vi "rechts.vi"   [LabVIEW 2019]
uses:
  <vilib>/myRIO/Common/Instrument Driver Framework/Utilities/typedefs/Analog Scaling Constants.ctl
  <vilib>/myRIO/Common/Instrument Driver Framework/Utilities/typedefs/Analog Scaling Constants List.ctl
  <vilib>/myRIO/Common/Instrument Driver Framework/myRIO v1.0/AO/typedefs/AO Channels Enum.ctl
  <vilib>/myRIO/Common/Instrument Driver Framework/myRIO v1.0/AO/typedefs/AO Channels List.ctl
  <vilib>/myRIO/Common/Instrument Driver Framework/Utilities/typedefs/Generic FPGA Reference.ctl
  <vilib>/myRIO/Common/Instrument Driver Framework/Utilities/typedefs/myRIO v1.0 Reference.ctl
  <vilib>/myRIO/Common/Instrument Driver Framework/Utilities/typedefs/Hardware Version Enum.ctl
  <vilib>/myRIO/Common/Instrument Driver Framework/Utilities/typedefs/myRIO Generic Hardware Reference.ctl
  <vilib>/myRIO/Instrument Drivers/Onboard IO/AO/typedefs/AO Reference.ctl
  <vilib>/myRIO/Instrument Drivers/Onboard IO/AO/AO.lvlib
  <vilib>/myRIO/Instrument Drivers/Onboard IO/AO/vis/Write.vi
  <vilib>/userDefined/High Color/nirio_resource_hc.ctl
  <vilib>/myRIO/Common/Instrument Driver Framework/myRIO v1.0/AO/vis/myRIO v1.1 Open AO.vi
  <vilib>/myRIO/Instrument Drivers/Onboard IO/AO/vis/myRIO AO Open.xnode
  <vilib>/myRIO/Common/Instrument Driver Framework/Utilities/vis/Is FPGA Ref Available.vi
  <vilib>/myRIO/Express VI/Onboard IO/AO/AO Express VI.xnode
  interface.vi
types:
  T1 = typedef "AO.lvlib/AO Reference.ctl" = cluster{"myRIO Reference":T2, "AO Channel List":T6, "AO Scaling Constant List":T8}
  T2 = typedef "myRIO Generic Hardware Reference.ctl" = cluster{"myRIO Model":T3, "myRIO Hardware Reference":T4}
  T3 = typedef "Hardware Version Enum.ctl" = enum16{"Unknown", "myRIO-1900", "myRIO-1950", "roboRIO", "NI ELVIS RIO CM", "ELVIS III"}
  T4 = typedef "myRIO v1.0 Reference.ctl" = cluster{"Generic FPGA Reference":T5, "Allow multiple opens":bool}
  T5 = typedef "Generic FPGA Reference.ctl" = refnum<k20>
  T6 = typedef "AO Channels List.ctl" = T7[]
  T7 = typedef "AO Channels Enum.ctl" = enum16{"Not Connected", "AudioOut/Left", "AudioOut/Right", "C/AO0", "C/AO1", "A/AO0", "A/AO1", "B/AO0", "B/AO1"}
  T8 = typedef "Analog Scaling Constants List.ctl" = T9[]
  T9 = typedef "Analog Scaling Constants.ctl" = cluster{"LSB Weight (Volts)":dbl, "Offset (Volts)":dbl, "Signed?":bool}
  T10 = typedef "nirio_resource_hc.ctl" = tag
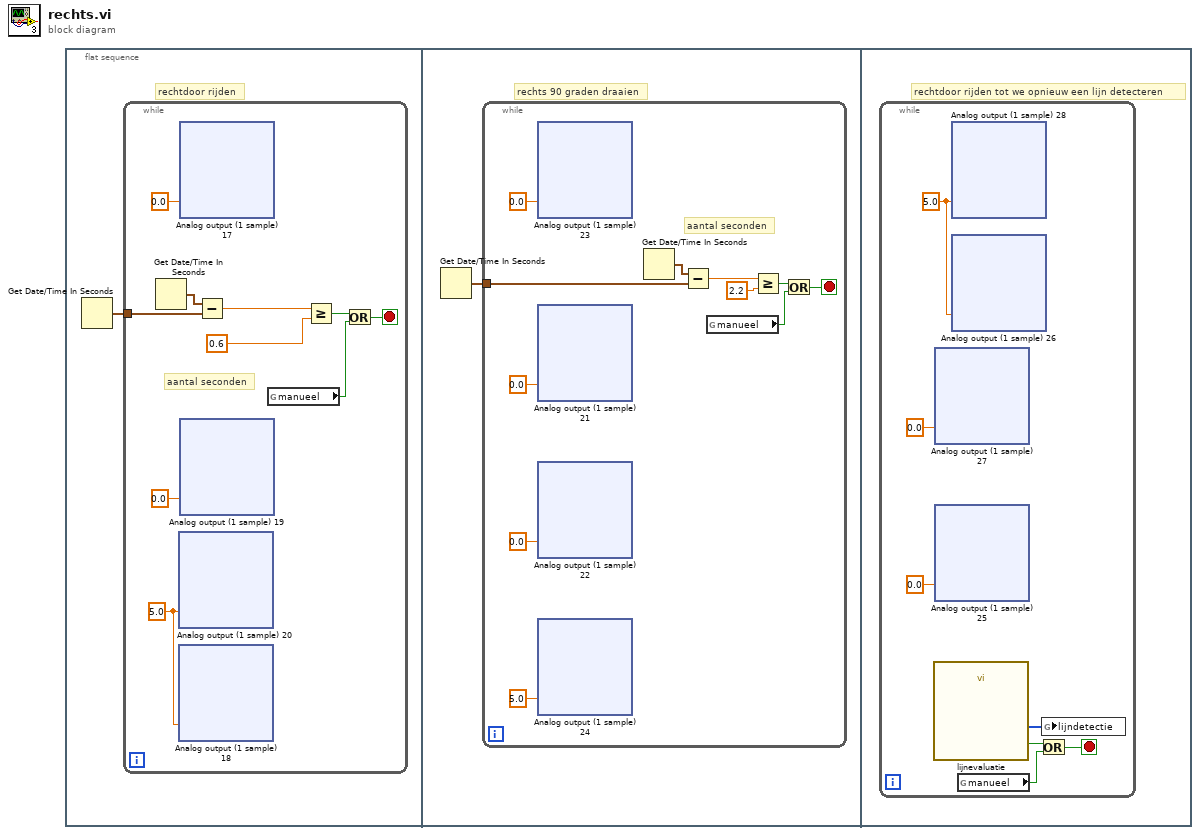
[diagram p0: block diagram]
diagram:
  n1 = flat-sequence {
    frame #0 {
      # "rechtdoor rijden"
      n2 = Get Date/Time In Seconds() -> (seconds since 1Jan1904=w1:timestamp)
      n3 = while {
        tunnel: w1 -> [w3]
        stop <- w7 stop-if-true
        w10 = 5.0
        # "aantal seconden"
        n4 = Get Date/Time In Seconds() -> (seconds since 1Jan1904=w5:timestamp)
        n5 = xnode "Analog output (1 sample) 20"("A/AO0 (Pin 2)"=w10) -> ()  [unwired: 1 in, 1 out]
        n6 = xnode "Analog output (1 sample) 18"("B/AO0 (Pin 2)"=w10) -> ()  [unwired: 1 in, 1 out]
        n7 = xnode "Analog output (1 sample) 17"("B/AO1 (Pin 4)"=0.0) -> ()  [unwired: 1 in, 1 out]
        n8 = xnode "Analog output (1 sample) 19"("A/AO1 (Pin 4)"=0.0) -> ()  [unwired: 1 in, 1 out]
        n9 = Subtract(x=w5, y=w3) -> (x-y=w6:dbl)
        n10 = global read "interface.vi" "manueel"() -> (w8:bool)
        n11 = Greater Or Equal?(x=w6, y=0.6) -> (x >= y?=w4:bool)
        n12 = Or(x=w4, y=w8) -> (x .or. y?=w7:bool)
      }
    }
    frame #1 {
      # "rechts 90 graden draaien"
      n13 = Get Date/Time In Seconds() -> (seconds since 1Jan1904=w160:timestamp)
      n14 = while {
        tunnel: w160 -> [w163]
        stop <- w166 stop-if-true
        # "aantal seconden"
        n15 = xnode "Analog output (1 sample) 23"("A/AO1 (Pin 4)"=0.0) -> ()  [unwired: 1 in, 1 out]
        n16 = xnode "Analog output (1 sample) 21"("B/AO1 (Pin 4)"=0.0) -> ()  [unwired: 1 in, 1 out]
        n17 = xnode "Analog output (1 sample) 22"("B/AO0 (Pin 2)"=0.0) -> ()  [unwired: 1 in, 1 out]
        n18 = xnode "Analog output (1 sample) 24"("A/AO0 (Pin 2)"=5.0) -> ()  [unwired: 1 in, 1 out]
        n19 = Get Date/Time In Seconds() -> (seconds since 1Jan1904=w164:timestamp)
        n20 = Subtract(x=w164, y=w163) -> (x-y=w165:dbl)
        n21 = global read "interface.vi" "manueel"() -> (w167:bool)
        n22 = Greater Or Equal?(x=w165, y=2.2) -> (x >= y?=w162:bool)
        n23 = Or(x=w162, y=w167) -> (x .or. y?=w166:bool)
      }
    }
    frame #2 {
      # "rechtdoor rijden tot we opnieuw een lijn detecteren"
      n24 = while {
        stop <- w323 stop-if-true
        w325 = 5.0
        n25 = call "lijnevaluatie.vi"() -> ("digitaal lijn 0-1"=w320:i32[], "lijn gedecteerd"=w321:bool)  [unwired: 8 in, 2 out]
        n26 = xnode "Analog output (1 sample) 27"("A/AO1 (Pin 4)"=0.0) -> ()  [unwired: 1 in, 1 out]
        n27 = xnode "Analog output (1 sample) 25"("B/AO1 (Pin 4)"=0.0) -> ()  [unwired: 1 in, 1 out]
        n28 = xnode "Analog output (1 sample) 28"("A/AO0 (Pin 2)"=w325) -> ()  [unwired: 1 in, 1 out]
        n29 = xnode "Analog output (1 sample) 26"("B/AO0 (Pin 2)"=w325) -> ()  [unwired: 1 in, 1 out]
        n30 = global read "interface.vi" "manueel"() -> (w322:bool)
        n31 = Or(x=w321, y=w322) -> (x .or. y?=w323:bool)
        n32 = global write "interface.vi" "lijndetectie"(w320) -> ()
      }
    }
  }
